vi "Action.vi"(8 "b":dbl, 10 "a":dbl, 11 "add in":refnum<class "add.lvclass">) -> (1 "result":dbl, 3 "add out":refnum<class "add.lvclass">)   [LabVIEW 2020, in "add.lvlib" / "add.lvclass"]
uses:
  add.lvclass
  add.lvclass/add.ctl
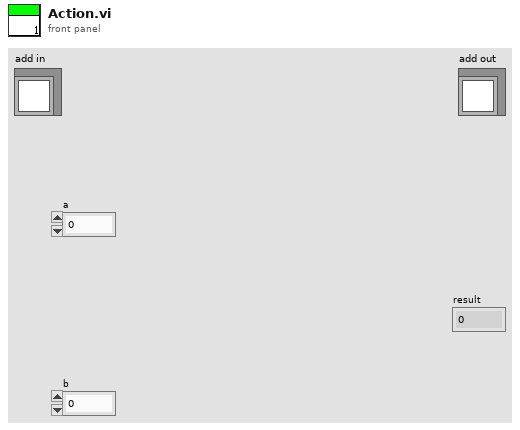
[diagram p1: front panel]
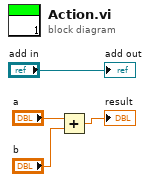
[diagram p0: block diagram]
diagram:
  n1 = Add(x="a", y="b") -> (x+y=→"result":dbl)
  "add out" <- "add in"
